vi "Configure Setpoint.vi"(0 "VISA resource name":refnum<visa-resource-name>, 5 "Loop (1:Loop 1)":u16(ring)=1 items=["Loop 1"=1, "Loop 2"=2], 7 "Setpoint Value (0.0000)":dbl format="%.4f", 11 "error in (no error)":errorcluster) -> (4 "VISA resource name out":refnum<visa-resource-name>, 15 "error out":errorcluster)   [LabVIEW 2019, in "Lake Shore 325.lvlib"]
doc: "This VI configures the control setpoint value. The control setpoint is the desired load temperature expressed in temperature or sensor units. Use sensor units if no temperature response curve is selected for the sensor input used as the control channel."
uses:
  <instrlib>/Lake Shore 325/Lake Shore 325.lvlib
  Instance           2 26Saved   Configure Setpoint .vi
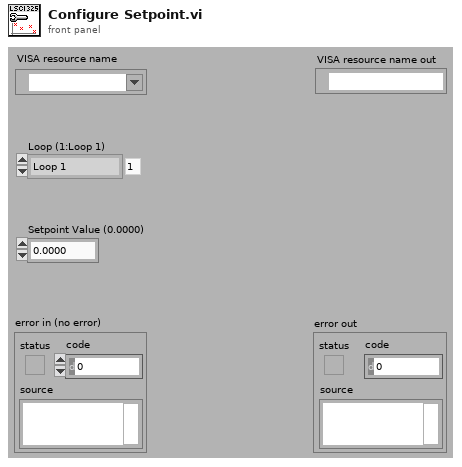
[diagram p1: front panel]
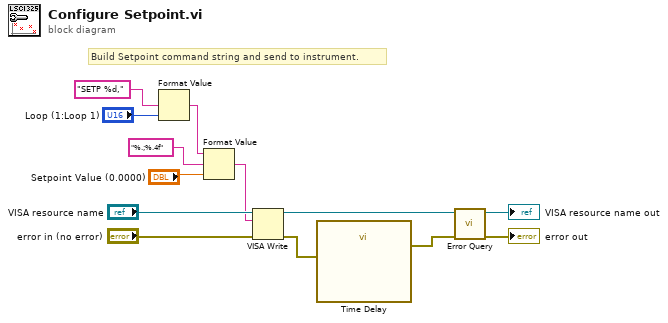
[diagram p0: block diagram]
diagram:
  # "Build Setpoint command string and send to instrument."
  n1 = Format Value(format string="SETP %d,", value (0)="Loop (1:Loop 1)") -> (output string=w3:string)  [unwired: 1 in]
  n2 = Format Value(string ("")=w3, format string="%.;%.4f", value (0)="Setpoint Value (0.0000)") -> (output string=w5:string)
  n3 = VISA Write(VISA resource name="VISA resource name", write buffer=w5, error in (no error)="error in (no error)") -> (VISA resource name out=w11:refnum<visa-resource-name>, error out=w2:errorcluster)  [unwired: 1 out]
  n4 = call "Time Delay"("error in (no error)"=w2) -> ("error out"=w1:errorcluster)  [unwired: 10 in]
  n5 = call <instrlib>:"Error Query.vi"("error in (no error)"=w1, "VISA resource name"=w11) -> ("error out"=→"error out":errorcluster, "VISA resource name out"=→"VISA resource name out":refnum<visa-resource-name>)  [unwired: 7 in, 1 out]
